vi "SSC DCPower Configure Output Enabled And Connected - Backup before Dec29 changes.vi"(0 "DCPower SSC in":T1[](array[typedef]), 5 "Output Enabled And Connected":bool, 11 "error in":errorcluster) -> (4 "DCPower SSC out":T1[](array[typedef]), 15 "error out":errorcluster)   [LabVIEW 2019]
doc: "This VI configures output enabled and connected on the channels.\n\nT - Enable and then connect\nF - Disconnect and then disable"
uses:
  SSC DCPower.ctl
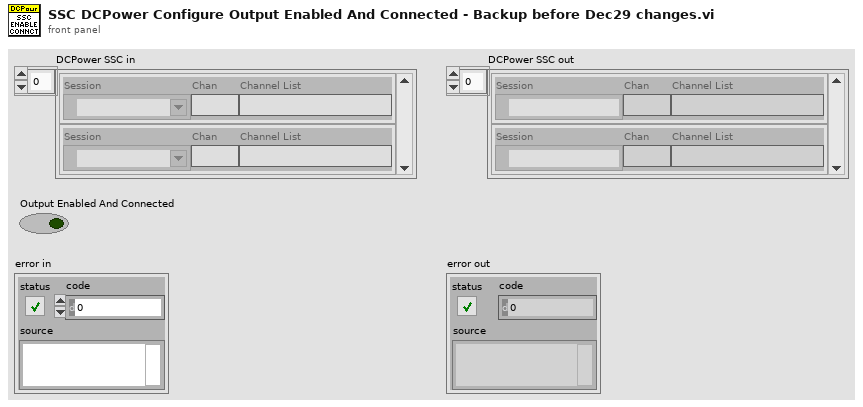
[diagram p1: front panel]
types:
  T1 = typedef "SSC DCPower.ctl" = cluster{"Session":refnum<k15>, "Chan":string, "Channel List":string}
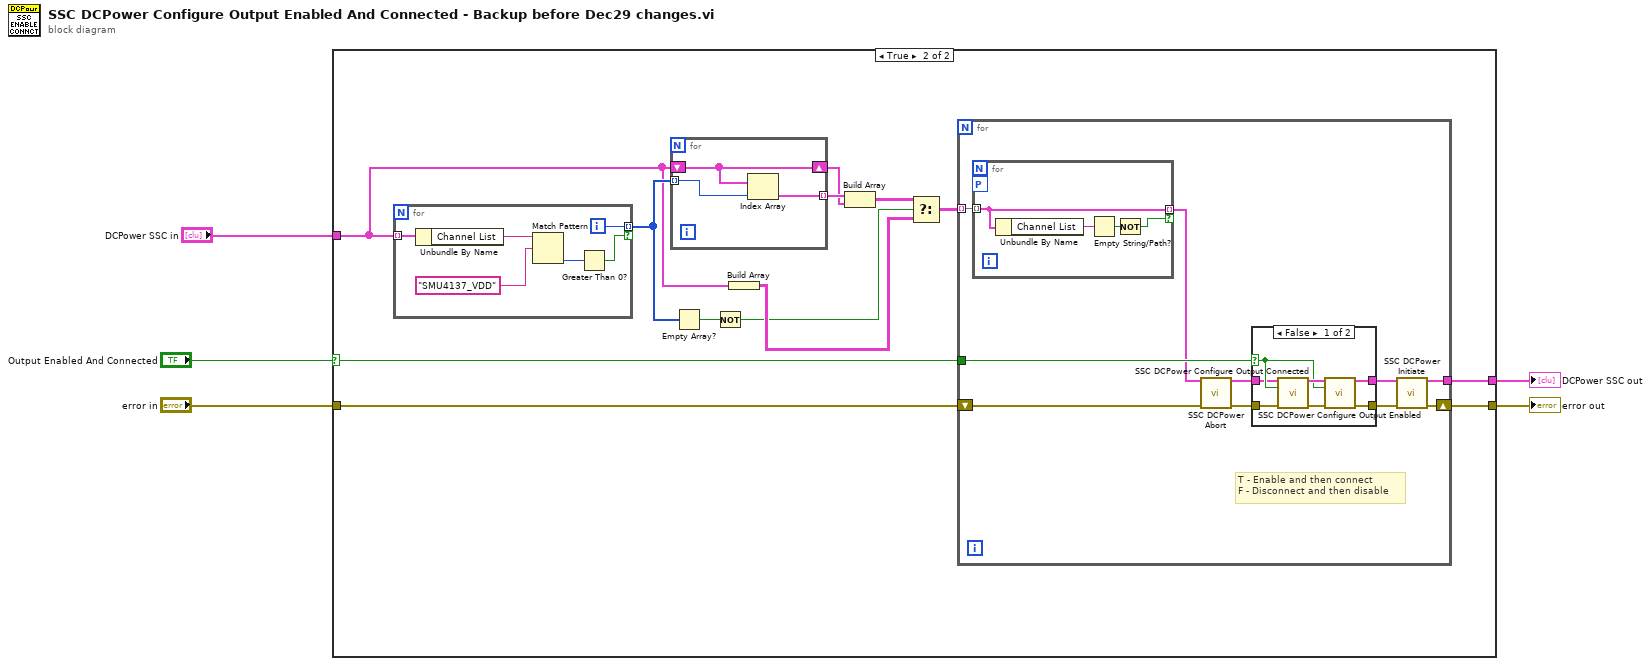
[diagram p0: block diagram]
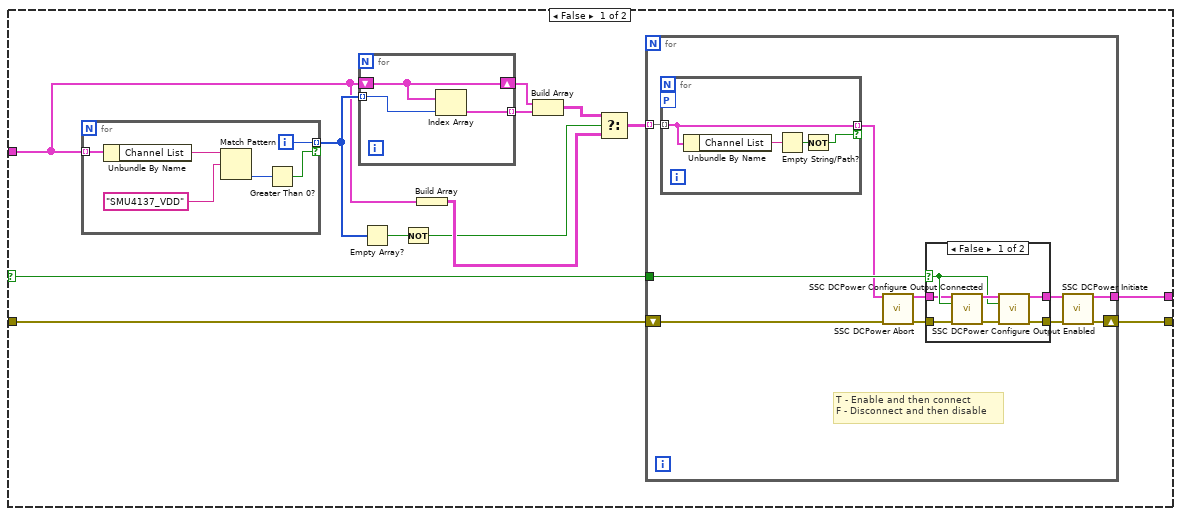
[diagram p2: hidden frame]
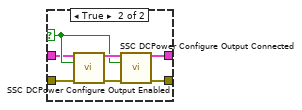
[diagram p3: hidden frame]
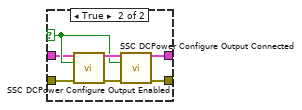
[diagram p4: hidden frame]
diagram:
  n1 = case shown="True" "Output Enabled And Connected" {
    selector: "Output Enabled And Connected" -> [w6 w56]
    tunnel: "error in" -> [w12 w68]
    tunnel: [w10 w67] -> w4
    tunnel: [w9 w66] -> w3
    tunnel: "DCPower SSC in" -> [w11 w60]
    frame False {
      n2 = for {
        tunnel: w11 -> [w27] mode=indexing
        tunnel: [w23] -> w18 mode=indexing if=w22
        i -> [w23]
        n3 = Unbundle By Name(w27) -> ("Channel List"=w26:string)
        n4 = Match Pattern(string=w26, regular expression="SMU4137_VDD") -> (offset past match=w24:i32)  [unwired: 1 in, 3 out]
        n5 = Greater Than 0?(x=w24) -> (x > 0?=w22:bool)
      }
      n6 = for {
        shift-right: [w20] -> w8
        shift-left: w11 -> [w20]
        tunnel: w18 -> [w21] mode=indexing
        tunnel: [w19] -> w7 mode=indexing
        n7 = Index Array(array=w20, index=w21) -> (element=w19:T1)
      }
      n8 = Empty Array?(array=w18) -> (empty?=w17:bool)
      n9 = Not(x=w17) -> (.not. x?=w14:bool)
      n10 = Build Array(w11) -> (w15:T1[][])
      n11 = Build Array(w8, w7) -> (w16:T1[][])
      n12 = Select(t=w16, s=w14, f=w15) -> (s? t:f=w13:T1[][])
      n13 = for {
        tunnel: [w28] -> w9
        tunnel: w6 -> [w37]
        shift-right: [w30] -> w10
        shift-left: w12 -> [w35]
        tunnel: w13 -> [w36] mode=indexing
        # "T - Enable and then connect\nF - Disconnect and then disable"
        n14 = for {
          tunnel: w36 -> [w41] mode=indexing
          workers-P: _ -> [_]
          tunnel: [w41] -> w33 mode=indexing if=w38
          n15 = Unbundle By Name(w41) -> ("Channel List"=w39:string)
          n16 = Empty String/Path?(string/path=w39) -> (empty?=w40:bool)
          n17 = Not(x=w40) -> (.not. x?=w38:bool)
        }
        n18 = call "SSC DCPower Abort.vi"("DCPower SSC in"=w33, "error in"=w35) -> ("DCPower SSC out"=w32:T1[], "error out"=w34:errorcluster)  [unwired: 12 in]
        n19 = case shown="False" w37 {
          selector: w37 -> [w43 w50]
          tunnel: w34 -> [w48 w55]
          tunnel: [w46 w53] -> w31
          tunnel: [w44 w51] -> w29
          tunnel: w32 -> [w42 w49]
          frame False {
            n20 = call "SSC DCPower Configure Output Connected.vi"("DCPower SSC in"=w42, "Output Connected"=w43, "error in"=w48) -> ("DCPower SSC out"=w45:T1[], "error out"=w47:errorcluster)  [unwired: 11 in]
            n21 = call "SSC DCPower Configure Output Enabled.vi"("DCPower SSC in"=w45, "Output Enabled"=w43, "error in"=w47) -> ("DCPower SSC out"=w44:T1[], "error out"=w46:errorcluster)  [unwired: 11 in]
          }
          frame True {
            n22 = call "SSC DCPower Configure Output Enabled.vi"("DCPower SSC in"=w49, "Output Enabled"=w50, "error in"=w55) -> ("DCPower SSC out"=w52:T1[], "error out"=w54:errorcluster)  [unwired: 11 in]
            n23 = call "SSC DCPower Configure Output Connected.vi"("DCPower SSC in"=w52, "Output Connected"=w50, "error in"=w54) -> ("DCPower SSC out"=w51:T1[], "error out"=w53:errorcluster)  [unwired: 11 in]
          }
        }
        n24 = call "SSC DCPower Initiate.vi"("DCPower SSC in"=w29, "error in"=w31) -> ("DCPower SSC out"=w28:T1[], "error out"=w30:errorcluster)  [unwired: 12 in]
      }
    }
    frame True {
      n25 = for {
        tunnel: w60 -> [w77] mode=indexing
        tunnel: [w73] -> w63 mode=indexing if=w72
        i -> [w73]
        n26 = Unbundle By Name(w77) -> ("Channel List"=w76:string)
        n27 = Match Pattern(string=w76, regular expression="SMU4137_VDD") -> (offset past match=w74:i32)  [unwired: 1 in, 3 out]
        n28 = Greater Than 0?(x=w74) -> (x > 0?=w72:bool)
      }
      n29 = for {
        shift-right: [w70] -> w64
        shift-left: w60 -> [w70]
        tunnel: w63 -> [w71] mode=indexing
        tunnel: [w69] -> w65 mode=indexing
        n30 = Index Array(array=w70, index=w71) -> (element=w69:T1)
      }
      n31 = Empty Array?(array=w63) -> (empty?=w62:bool)
      n32 = Not(x=w62) -> (.not. x?=w58:bool)
      n33 = Build Array(w60) -> (w59:T1[][])
      n34 = Build Array(w65, w64) -> (w61:T1[][])
      n35 = Select(t=w61, s=w58, f=w59) -> (s? t:f=w57:T1[][])
      n36 = for {
        tunnel: [w79] -> w66
        tunnel: w56 -> [w87]
        shift-right: [w78] -> w67
        shift-left: w68 -> [w85]
        tunnel: w57 -> [w86] mode=indexing
        # "T - Enable and then connect\nF - Disconnect and then disable"
        n37 = for {
          tunnel: w86 -> [w91] mode=indexing
          workers-P: _ -> [_]
          tunnel: [w91] -> w84 mode=indexing if=w88
          n38 = Unbundle By Name(w91) -> ("Channel List"=w89:string)
          n39 = Empty String/Path?(string/path=w89) -> (empty?=w90:bool)
          n40 = Not(x=w90) -> (.not. x?=w88:bool)
        }
        n41 = call "SSC DCPower Abort.vi"("DCPower SSC in"=w84, "error in"=w85) -> ("DCPower SSC out"=w82:T1[], "error out"=w83:errorcluster)  [unwired: 12 in]
        n42 = case shown="False" w87 {
          selector: w87 -> [w93 w100]
          tunnel: w83 -> [w98 w105]
          tunnel: [w96 w103] -> w81
          tunnel: [w94 w101] -> w80
          tunnel: w82 -> [w92 w99]
          frame False {
            n43 = call "SSC DCPower Configure Output Connected.vi"("DCPower SSC in"=w92, "Output Connected"=w93, "error in"=w98) -> ("DCPower SSC out"=w95:T1[], "error out"=w97:errorcluster)  [unwired: 11 in]
            n44 = call "SSC DCPower Configure Output Enabled.vi"("DCPower SSC in"=w95, "Output Enabled"=w93, "error in"=w97) -> ("DCPower SSC out"=w94:T1[], "error out"=w96:errorcluster)  [unwired: 11 in]
          }
          frame True {
            n45 = call "SSC DCPower Configure Output Enabled.vi"("DCPower SSC in"=w99, "Output Enabled"=w100, "error in"=w105) -> ("DCPower SSC out"=w102:T1[], "error out"=w104:errorcluster)  [unwired: 11 in]
            n46 = call "SSC DCPower Configure Output Connected.vi"("DCPower SSC in"=w102, "Output Connected"=w100, "error in"=w104) -> ("DCPower SSC out"=w101:T1[], "error out"=w103:errorcluster)  [unwired: 11 in]
          }
        }
        n47 = call "SSC DCPower Initiate.vi"("DCPower SSC in"=w80, "error in"=w81) -> ("DCPower SSC out"=w79:T1[], "error out"=w78:errorcluster)  [unwired: 12 in]
      }
    }
  }
  "error out" <- w4
  "DCPower SSC out" <- w3
